vi "8switches.vi"() -> ()   [LabVIEW 2017]
panel:
  in  "Array 2":bool[](array[boolean])
  out "Array":bool[](array[boolean])
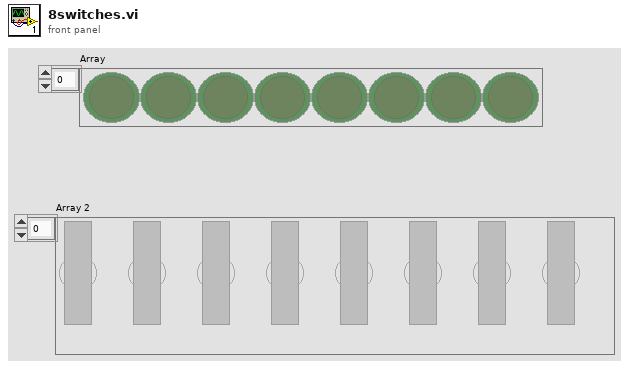
[diagram p1: front panel]
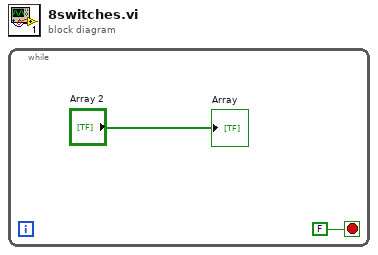
[diagram p0: block diagram]
diagram:
  n1 = while {
    stop <- FALSE stop-if-true
    "Array" <- "Array 2"
  }
